vi "State_Machine.vi"(8 "error in (no error)":errorcluster caption="entrée d'erreur (pas d'erreur)", 11 "Check_Func en entrée":refnum<class "Check_Func.lvclass">) -> (0 "error out":errorcluster caption="sortie d'erreur", 2 "Json_String":string, 3 "Check_Func en sortie":refnum<class "Check_Func.lvclass">)   [LabVIEW 2020, in "Library Test.lvlib" / "Check_Func.lvclass"]
uses:
  Check_Func.lvclass
  Check_Func.lvclass/Check_Func.ctl
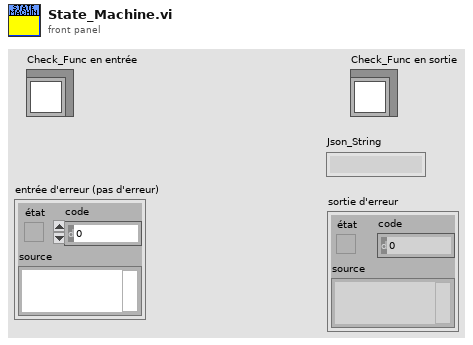
[diagram p1: front panel]
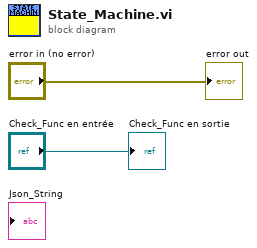
[diagram p0: block diagram]
diagram:
  "Check_Func en sortie" <- "Check_Func en entrée"
  "error out" <- "error in (no error)"
